vi "Get Trigger Channels.vi"(8 "error in":errorcluster, 11 "acyclic frames section in":T1 format="%.0x") -> (0 "error out":errorcluster, 2 "acyclic frame triggers":T1[](array[typedef]) format="%.0x", 3 "acyclic frames section out":T1 format="%.0x", 4 "found?":bool)   [LabVIEW 2020, in "AIM MIL-STD-1553 Scripting.lvlib"]
uses:
  AIM MIL-STD-1553 Scripting.lvlib
  <vilib>/NI VeriStand/Custom Device API/Custom Device Item Ref.ctl
  Constants.vi
  <vilib>/NI VeriStand/Custom Device Tools/Custom Device Utility Library/NI VeriStand - Search for All Items by GUID.vi
  <vilib>/NI VeriStand/Custom Device Tools/Custom Device Utility Library/Custom Device Utility Library.lvlib
  <vilib>/NI VeriStand/Custom Device API/Custom Device API.lvlib
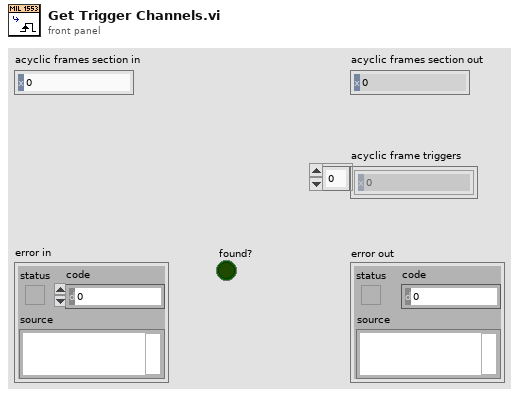
[diagram p1: front panel]
types:
  T1 = typedef "Custom Device API.lvlib/Custom Device Item Ref.ctl" = u64
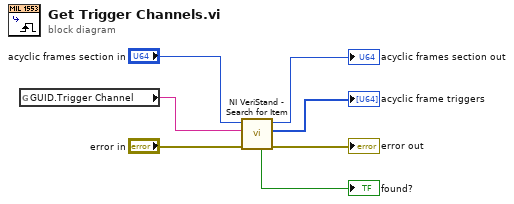
[diagram p0: block diagram]
diagram:
  n1 = global read "Constants.vi" "GUID.Trigger Channel"() -> (w4:string)
  n2 = call-poly <vilib>:"NI VeriStand - Search for Item.vi"("error in"="error in", "Item GUID"=w4, "Section Ref in"="acyclic frames section in") -> ("error out"=→"error out":errorcluster, "Item Refs"=→"acyclic frame triggers":T1[], "Section Ref out"=→"acyclic frames section out":T1, "Found"=→"found?":bool)  [unwired: 5 in]
